vi "RT Watchdog Setup.vi"(8 "error in (no error)":errorcluster) -> (0 "error out":errorcluster, 3 "watchdogID":u64)   [LabVIEW 2017]
doc: "Author: Scott Hannahs <sth@magnet.fsu.edu>\nCopyright 2018 Florida State University, All rights reserved."
uses:
  <vilib>/RTwatchdog.llb/Watchdog expiration actions.ctl
panel:
  out "timeout value returned (sec)":dbl format="%^.2e"
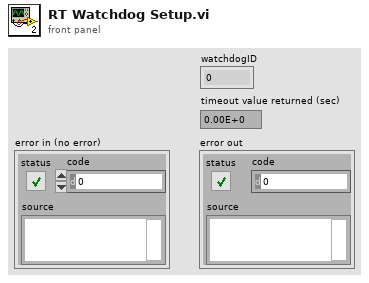
[diagram p1: front panel]
types:
  T1 = typedef "Watchdog expiration actions.ctl" = cluster{"reset system":bool, "restart LabVIEW Runtime":bool, "occurrence":bool, "trigger protocol":enum16{"active high", "active low", "open collector"}, "trigger line":enum16{"none", "line 0", "line 1", "line 2", "line 3", "line 4", "line 5", "line 6", "line 7", "SMB line 0"}, "disable watchdog on VI exit":bool}
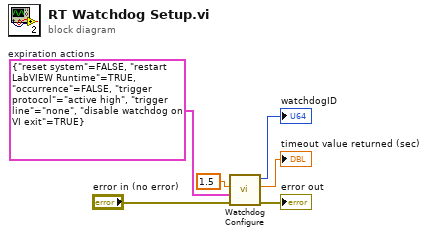
[diagram p0: block diagram]
diagram:
  w2 = T1 {"reset system"=FALSE, "restart LabVIEW Runtime"=TRUE, "occurrence"=FALSE, "trigger protocol"=enum."active high", "trigger line"=enum."none", "disable watchdog on VI exit"=TRUE}  # expiration actions
  n1 = call <vilib>:"Watchdog Configure.vi"("error in (no error)"="error in (no error)", "expiration actions"=w2, "timeout (1 sec)"=1.5) -> ("error out"=→"error out":errorcluster, "timeout value returned (sec)"=→"timeout value returned (sec)":dbl, "watchdogID"=→"watchdogID":u64)  [unwired: 1 in, 1 out]
